vi "Write INIndex.vi"(8 "error in (no error)":errorcluster, 10 "INIndex":i32, 11 "LineScan in":refnum<class "LineScan.lvclass">) -> (0 "error out":errorcluster, 3 "LineScan out":refnum<class "LineScan.lvclass">)   [LabVIEW 2019, in "LineScan.lvclass"]
uses:
  LineScan.lvclass
  Ctrl/Auto Inspection_IN Name.ctl
  FlowIOCtrl.lvclass
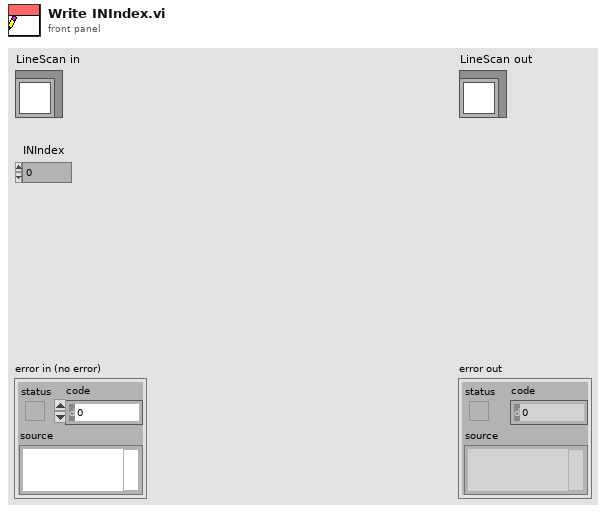
[diagram p1: front panel]
types:
  T1 = typedef "Auto Inspection_IN Name.ctl" = enum16{"ItemInWorkPos", "ItemReadyIn", "ItemInSensor", "StopUpSensor", "SlowSensor", "TrayUp", "Fix", "Release fix", "TrayDown", "NextRequest", "StopDown", "ConveyorOut"}
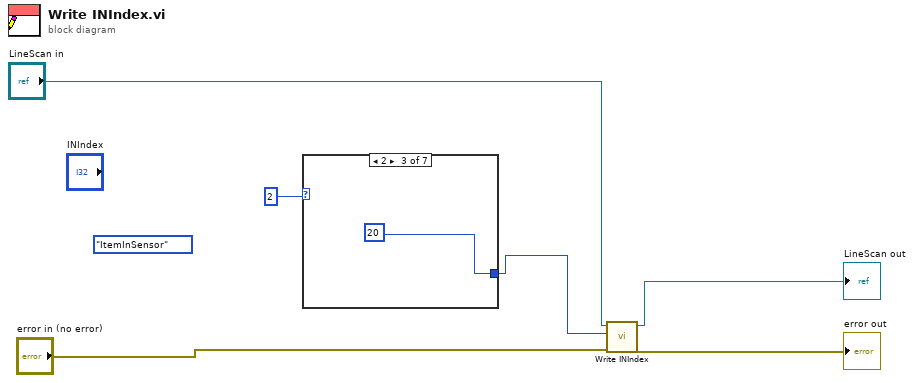
[diagram p0: block diagram]
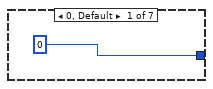
[diagram p2: hidden frame]
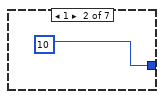
[diagram p3: hidden frame]
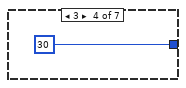
[diagram p4: hidden frame]
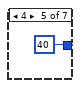
[diagram p5: hidden frame]
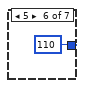
[diagram p6: hidden frame]
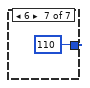
[diagram p7: hidden frame]
diagram:
  (unwired) Auto_Inspection_IN_Name."ItemInSensor"
  n1 = case shown="2" 2 {
    tunnel: [0 10 20 30 40 110 110 ("ModbusIOInput")] -> w2
    frame 0, Default {
    }
    frame 1 {
    }
    frame 2 {
    }
    frame 3 {
    }
    frame 4 {
    }
    frame 5 {
    }
    frame 6 {
    }
  }
  n2 = call-parent "Write INIndex.vi"("error in (no error)"="error in (no error)", "INIndex"=w2, "Station Action in"="LineScan in") -> ("error out"=→"error out":errorcluster, "Station Action out"=→"LineScan out":refnum<class "LineScan.lvclass">)  [unwired: 7 in]
